vi "DAQmx 9481 4ch Relay (SubVI).vi"(0 "9481 Name":tag="9481", 7 "Relay Control":bool[](array[boolean])=[FALSE, FALSE, FALSE, FALSE], 11 "Error Input":errorcluster, 13 "Stop Program":bool) -> (15 "9481 Error":errorcluster)   [LabVIEW 2012]
uses:
  <vilib>/DAQmx/write.llb/DAQmx Write (Digital 1D Bool NChan 1Samp 1Line).vi
  <vilib>/DAQmx/create/channels.llb/DAQmx Create Channel (DO-Digital Output).vi
  <vilib>/DAQmx/miscellaneous.llb/DAQmx Fill In Error Info.vi
panel:
  # "DAQmx - 9481\n4ch Relay\nCreated by Blake Otting \nLast Update 11-15-2012"
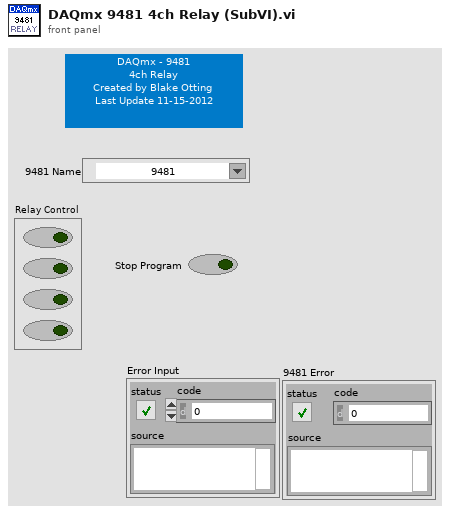
[diagram p1: front panel]
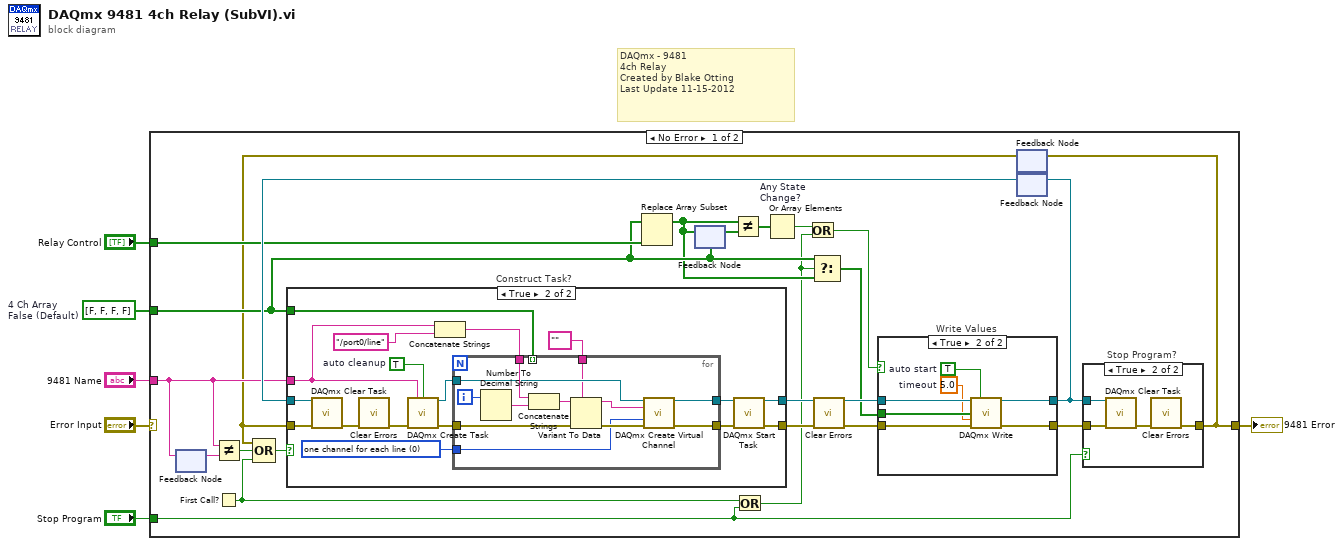
[diagram p0: block diagram]
diagram:
  w3 = bool[] [FALSE, FALSE, FALSE, FALSE]  # 4 Ch Array False (Default)
  # "DAQmx - 9481\n4ch Relay\nCreated by Blake Otting \nLast Update 11-15-2012"
  n1 = case shown="No Error" "Error Input" {
    selector: "Error Input" -> [_ w75]
    tunnel: "Relay Control" -> [w22 _]
    tunnel: [w28 w75] -> w2
    tunnel: "9481 Name" -> [w12 _]
    tunnel: "Stop Program" -> [w16 _]
    tunnel: w3 -> [w19 _]
    frame No Error {
      n2 = feedback-in #1(w12) -> ()
      n3 = feedback #1() -> (w11:tag)  [unwired: 1 in]
      n4 = Not Equal?(x=w12, y=w11) -> (x != y?=w9:bool)
      n5 = First Call?() -> (First Call?: T/F=w8:bool)
      n6 = Replace Array Subset(array=w19, new element=w22) -> (w18:bool[])  [unwired: 1 in]
      n7 = feedback-in #2(w18) -> ()
      n8 = feedback #2(w19) -> (w21:bool[])
      n9 = Not Equal?(x=w18, y=w21) -> (x != y?=w20:bool[])
      n10 = Or(x=w8, y=w16) -> (x .or. y?=w14:bool)
      n11 = Or Array Elements "Any State\nChange?"(Boolean array=w20) -> (logical OR=w15:bool)
      n12 = Or(x=w15, y=w14) -> (x .or. y?=w13:bool)
      n13 = Select(t=w19, s=w14, f=w18) -> (s? t:f=w17:bool[])
      n14 = feedback #3() -> (w10:errorcluster)  [unwired: 1 in]
      n15 = Compound Arithmetic op=OR(w10, w9, w8) -> (w7:bool)
      n16 = feedback #4() -> (w26:refnum<k21>)  [unwired: 1 in]
      n17 = case "Construct Task?" shown="True" w7 {
        tunnel: [w40 w48] -> w25
        tunnel: [w39 w47] -> w24
        tunnel: w10 -> [w39 w52]
        tunnel: w26 -> [w40 w53]
        tunnel: w12 -> [_ w43]
        tunnel: w19 -> [_ w41]
        frame False {
        }
        frame True {
          w56 = 0 items=["one channel for each line", "one channel for all lines"]
          w57 = TRUE  # auto cleanup
          n18 = call <vilib>:"DAQmx Clear Task.vi"("task in"=w53, "error in"=w52) -> ("error out"=w51:errorcluster)  [unwired: 13 in]
          n19 = call <vilib>:"Clear Errors.vi"("error in (no error)"=w51) -> ("error out"=w50:errorcluster)  [unwired: 6 in]
          n20 = call <vilib>:"DAQmx Create Task.vi"("new task name"=w43, "auto cleanup"=w57, "error in"=w50) -> ("task out"=w54:refnum<k21>, "error out"=w55:errorcluster)  [unwired: 11 in]
          n21 = Concatenate Strings(w43, "/port0/line" ("string")) -> (w46:string)
          n22 = for {
            tunnel: w46 -> [w67]
            tunnel: w55 -> [w66]
            tunnel: [w60] -> w44
            tunnel: w54 -> [w62]
            tunnel: [w61] -> w45
            tunnel: w56 -> [w59]
            tunnel: tag "" ("physical channels") -> [w58]
            tunnel: w41 -> [_] mode=indexing
            i -> [w68]
            n23 = Number To Decimal String(number=w68) -> (decimal integer string=w69:string)  [unwired: 1 in]
            n24 = Concatenate Strings(w67, w69) -> (w63:string)
            n25 = Variant To Data(error in=w66, type=w58, Variant=w63) -> (data=w64:tag, error out=w65:errorcluster)
            n26 = call-poly <vilib>:"DAQmx Create Virtual Channel.vi"("task in"=w62, "lines"=w64, "line grouping"=w59, "error in"=w65) -> ("task out"=w61:refnum<k21>, "error out"=w60:errorcluster)  [unwired: 10 in]
          }
          n27 = call <vilib>:"DAQmx Start Task.vi"("task/channels in"=w45, "error in"=w44) -> ("task out"=w48:refnum<k21>, "error out"=w47:errorcluster)  [unwired: 12 in]
        }
      }
      n28 = call <vilib>:"Clear Errors.vi"("error in (no error)"=w24) -> ("error out"=w23:errorcluster)  [unwired: 6 in]
      n29 = case "Write Values" shown="True" w13 {
        tunnel: w25 -> [w31 w37]
        tunnel: w23 -> [w30 w36]
        tunnel: w17 -> [_ w35]
        tunnel: [w30 w34] -> w29
        tunnel: [w31 w32] -> w27
        frame False {
        }
        frame True {
          w33 = 5.0  # timeout
          w38 = TRUE  # auto start
          n30 = call-poly <vilib>:"DAQmx Write.vi"("task/channels in"=w37, "auto start"=w38, "data"=w35, "timeout"=w33, "error in"=w36) -> ("task out"=w32:refnum<k21>, "error out"=w34:errorcluster)  [unwired: 8 in, 1 out]
        }
      }
      n31 = feedback-in #4(w27) -> ()
      n32 = case "Stop Program?" shown="True" w16 {
        tunnel: w27 -> [_ w72]
        tunnel: w29 -> [w70 w73]
        tunnel: [w70 w71] -> w28
        frame False {
        }
        frame True {
          n33 = call <vilib>:"DAQmx Clear Task.vi"("task in"=w72, "error in"=w73) -> ("error out"=w74:errorcluster)  [unwired: 13 in]
          n34 = call <vilib>:"Clear Errors.vi"("error in (no error)"=w74) -> ("error out"=w71:errorcluster)  [unwired: 6 in]
        }
      }
      n35 = feedback-in #3(w28) -> ()
    }
    frame Error {
    }
  }
  "9481 Error" <- w2
